vi "destroy.vi"(8 "error in (no error)":errorcluster, 11 "MsgUserEventStopMechanism In":refnum<class "MsgQueueTaskChannel.lvclass">) -> (0 "error out":errorcluster, 3 "MsgUserEventStopMechanism Out":refnum<class "MsgQueueTaskChannel.lvclass">)   [LabVIEW 2023, in "TLC_Daemon.lvlib" / "MsgQueueTaskChannel.lvclass"]
doc: "Destroy procedure"
uses:
  MsgUETaskChannel/MsgQueueTaskChannel.lvclass
  MsgUETaskChannel/MsgQueueTaskChannel.lvclass/MsgQueueTaskChannel.ctl
  Ctrls/msg.ctl
  TLC_Daemon.lvlib
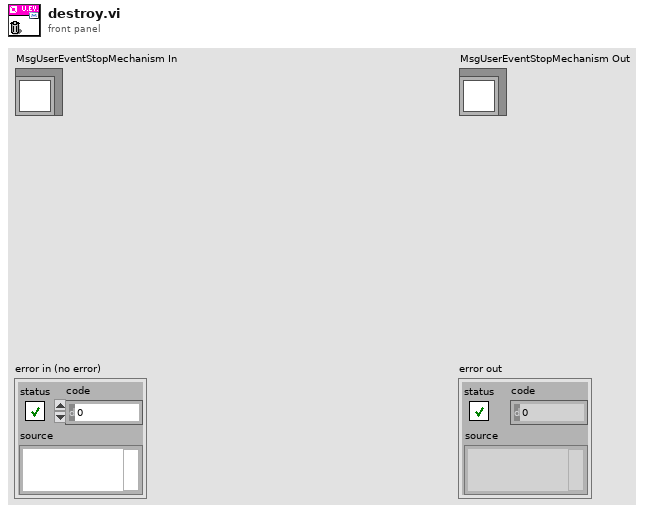
[diagram p1: front panel]
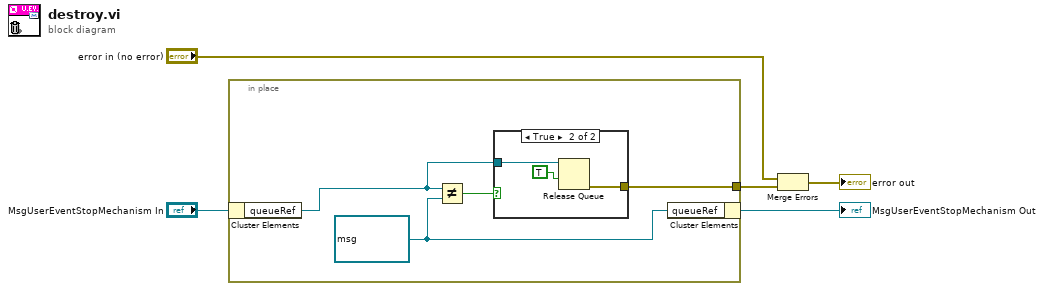
[diagram p0: block diagram]
diagram:
  n1 = in-place {
    in-place-border: [w7] -> w2
    w6 = refnum<queue> refnum ("queueRef")
    n2 = in-place-cluster #1("MsgUserEventStopMechanism In") -> ("queueRef"=w8:refnum<queue>)
    n3 = Not Equal?(x=w8, y=w6) -> (x != y?=w9:bool)
    n4 = case shown="True" w9 {
      tunnel: w8 -> [_ w12]
      tunnel: [_ w11] -> w7
      frame False {
      }
      frame True {
        n5 = Release Queue(queue=w12, force destroy? (F)=TRUE) -> (error out=w11:errorcluster)  [unwired: 1 in, 2 out]
      }
    }
    n6 = in-place-cluster #1("queueRef"=w6) -> (→"MsgUserEventStopMechanism Out":refnum<class "MsgQueueTaskChannel.lvclass">)
  }
  n7 = Merge Errors("error in (no error)", w2) -> (→"error out":errorcluster)
